vi "Total Names.vi"(7 "Include Suffix":bool, 10 "Contol\nPoint\nSuffix":T1) -> (2 "Names":string[](array[string]))   [LabVIEW 2009]
uses:
  Name Actions.ctl
  NTCP Client/Control Point Suffix.ctl
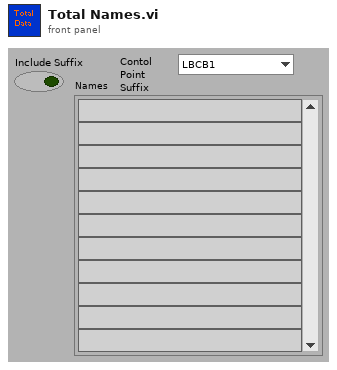
[diagram p1: front panel]
types:
  T1 = typedef "Control Point Suffix.ctl" = enum16{"LBCB1", "LBCB2", "ExternalSensors"}
  T2 = typedef "Name Actions.ctl" = enum16{"Init", "Get Names", "Get Index"}
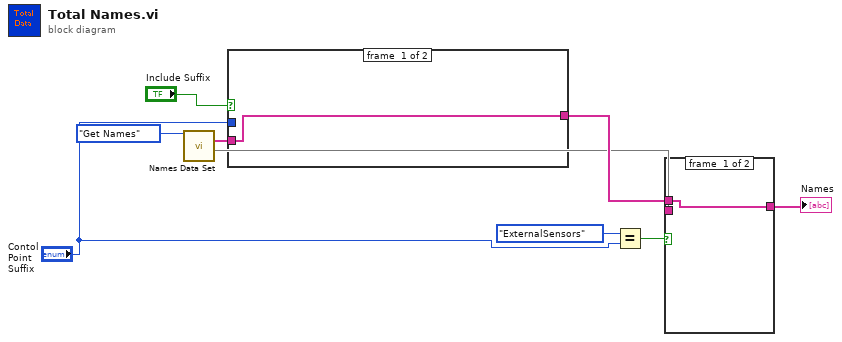
[diagram p0: block diagram]
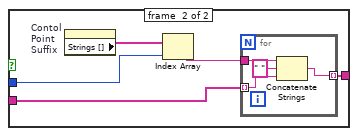
[diagram p2: hidden frame]
diagram:
  n1 = call "Names Data Set.vi"("Name Actions"=Name_Actions."Get Names") -> ("Cartesian Readings"=w7:string[], 12:w5)  [unwired: 1 in, 12 out]
  n2 = case shown="True" "Include Suffix" {
    tunnel: [w10 w13] -> w8
    tunnel: w7 -> [w10 w12]
    tunnel: "Contol\nPoint\nSuffix" -> [_ w11]
    frame #0 {
    }
    frame #1 {
      n3 = property on="Contol\nPoint\nSuffix" class="Enum (strict)"() -> ("Strings []"=w15:string[])  [unwired: 2 in, 2 out]
      n4 = Index Array(array=w15, index=w11) -> (element=w14:string)
      n5 = for {
        tunnel: w14 -> [w19]
        tunnel: w12 -> [w17] mode=indexing
        tunnel: [w18] -> w13 mode=indexing
        n6 = Concatenate Strings(w19, " " ("string"), w17) -> (w18:string)
      }
    }
  }
  n7 = Equal?(x=Control_Point_Suffix."ExternalSensors", y="Contol\nPoint\nSuffix") -> (x = y?=w4:bool)
  n8 = case shown="True" w4 {
    tunnel: w8 -> [w20 _]
    tunnel: [w20 w21] -> w6
    tunnel: w5 -> [_ w21]
    frame #0 {
    }
    frame #1 {
    }
  }
  "Names" <- w6
